vi "gyro -- async pll monitor V1.vi"(11 "pll monitor event pair IN":T6) -> ()   [LabVIEW 2020]
uses:
  lorentzian.ctl
  circle corners.ctl
  show-win- control.ctl
  server talk-to-back pair.ctl
  server talkback message type.ctl
  server talkto message type.ctl
  interpolation state - real.ctl
  pll internal user event action.ctl
  launch items list.ctl
  que event bag action.ctl
  agregator -- action.ctl
  interpolation state - complex.ctl
  publisher action.ctl
  cursor action.ctl
  four-corner circle transformation.ctl
  linear interpolation iiii- complex.vi
  replace cursor action stack.vi
  Q -- range multiplier -- real -- V2.vi
  Q - not nan and gtr than zero - Real.vi
  Q - not nan -- real.vi
  Q -- check range -- i -- real.vi
  array - smart min max.vi
  linear interpolation - real.vi
  draw a circle.vi
  draw a complex arrow.vi
  generate linear region.vi
  draw a complex line.vi
panel:
  in  "all 3":T1(tab)
  in  "Reset lore :q":bool
  in  "Tab Control":enum32{"PID", "hist", "params"}(tab)
  out "Plot: complex plane":cluster{dbl[], dbl[]}[](graph)=[{[0.0, 0.0, 0.0, 0.0, 0.0, 0.0, 0.0, 0.0, 0.0, 0.0, 0.0, 0.0, 0.0, 0.0, 0.0, 0.0, 0.0, 0.0, 0.0, 0.0, 0.0, 0.0, 0.0, 0.0, 0.0, 0.0, 0.0, 0.0, 0.0, 0.0, 0.0, 0.0, 0.0, 0.0, 0.0, 0.0, 0.0, 0.0, 0.0, 0.0, 0.0, 0.0, 0.0, 0.0, 0.0, 0.0, 0.0, 0.0, 0.0, 0.0, 0.0, 0.0, 0.0, 0.0, 0.0, 0.0, 0.0, 0.0, 0.0, 0.0, 0.0, 0.0, 0.0, 0.0, 0.0, 0.0, 0.0, 0.0, 0.0, 0.0, 0.0, 0.0, 0.0, 0.0, 0.0, 0.0, 0.0, 0.0, 0.0, 0.0, 0.0, 0.0, 0.0, 0.0, 0.0, 0.0, 0.0, 0.0, 0.0, 0.0, 0.0, 0.0, 0.0, 0.0, 0.0, 0.0, 0.0, 0.0, 0.0, 0.0, 0.0, 0.0, 0.0, 0.0, 0.0, 0.0, 0.0, 0.0, 0.0, 0.0, 0.0, 0.0, 0.0, 0.0, 0.0, 0.0, 0.0, 0.0, 0.0, 0.0, 0.0, 0.0, 0.0, 0.0, 0.0, 0.0, 0.0, 0.0, 0.0, 0.0, 0.0, 0.0, 0.0, 0.0, 0.0, 0.0, 0.0, 0.0, 0.0, 0.0, 0.0, 0.0, 0.0, 0.0, 0.0, 0.0, 0.0, 0.0, 0.0, 0.0], [0.0, 0.0, 0.0, 0.0, 0.0, 0.0, 0.0, 0.0, 0.0, 0.0, 0.0, 0.0, 0.0, 0.0, 0.0, 0.0, 0.0, 0.0, 0.0, 0.0, 0.0, 0.0, 0.0, 0.0, 0.0, 0.0, 0.0, 0.0, 0.0, 0.0, 0.0, 0.0, 0.0, 0.0, 0.0, 0.0, 0.0, 0.0, 0.0, 0.0, 0.0, 0.0, 0.0, 0.0, 0.0, 0.0, 0.0, 0.0, 0.0, 0.0, 0.0, 0.0, 0.0, 0.0, 0.0, 0.0, 0.0, 0.0, 0.0, 0.0, 0.0, 0.0, 0.0, 0.0, 0.0, 0.0, 0.0, 0.0, 0.0, 0.0, 0.0, 0.0, 0.0, 0.0, 0.0, 0.0, 0.0, 0.0, 0.0, 0.0, 0.0, 0.0, 0.0, 0.0, 0.0, 0.0, 0.0, 0.0, 0.0, 0.0, 0.0, 0.0, 0.0, 0.0, 0.0, 0.0, 0.0, 0.0, 0.0, 0.0, 0.0, 0.0, 0.0, 0.0, 0.0, 0.0, 0.0, 0.0, 0.0, 0.0, 0.0, 0.0, 0.0, 0.0, 0.0, 0.0, 0.0, 0.0, 0.0, 0.0, 0.0, 0.0, 0.0, 0.0, 0.0, 0.0, 0.0, 0.0, 0.0, 0.0, 0.0, 0.0, 0.0, 0.0, 0.0, 0.0, 0.0, 0.0, 0.0, 0.0, 0.0, 0.0, 0.0, 0.0, 0.0, 0.0, 0.0, 0.0, 0.0, 0.0]}, {[0.0, 0.0, 0.0, 0.0, 0.0, 0.0, 0.0, 0.0, 0.0, 0.0, 0.0, 0.0, 0.0, 0.0, 0.0, 0.0, 0.0, 0.0, 0.0, 0.0], [0.0, 0.0, 0.0, 0.0, 0.0, 0.0, 0.0, 0.0, 0.0, 0.0, 0.0, 0.0, 0.0, 0.0, 0.0, 0.0, 0.0, 0.0, 0.0, 0.0]}, {[0.0, 0.0, 0.0, 0.0, 0.0, 0.0, 0.0, 0.0, 0.0, 0.0, 0.0, 0.0, 0.0, 0.0, 0.0, 0.0, 0.0, 0.0, 0.0, 0.0], [0.0, 0.0, 0.0, 0.0, 0.0, 0.0, 0.0, 0.0, 0.0, 0.0, 0.0, 0.0, 0.0, 0.0, 0.0, 0.0, 0.0, 0.0, 0.0, 0.0]}, {[0.0, 0.0, 0.0, 0.0, 0.0, 0.0, 0.0, 0.0, 0.0, 0.0, 0.0, 0.0, 0.0, 0.0, 0.0, 0.0, 0.0, 0.0, 0.0, 0.0], [0.0, 0.0, 0.0, 0.0, 0.0, 0.0, 0.0, 0.0, 0.0, 0.0, 0.0, 0.0, 0.0, 0.0, 0.0, 0.0, 0.0, 0.0, 0.0, 0.0]}, {[0.0, 0.0, 0.0, 0.0, 0.0, 0.0, 0.0, 0.0, 0.0, 0.0, 0.0, 0.0, 0.0, 0.0, 0.0, 0.0, 0.0, 0.0, 0.0, 0.0], [0.0, 0.0, 0.0, 0.0, 0.0, 0.0, 0.0, 0.0, 0.0, 0.0, 0.0, 0.0, 0.0, 0.0, 0.0, 0.0, 0.0, 0.0, 0.0, 0.0]}, {[0.0, 0.0, 0.0, 0.0, 0.0, 0.0, 0.0, 0.0, 0.0, 0.0, 0.0, 0.0, 0.0, 0.0, 0.0, 0.0, 0.0, 0.0, 0.0, 0.0], [0.0, 0.0, 0.0, 0.0, 0.0, 0.0, 0.0, 0.0, 0.0, 0.0, 0.0, 0.0, 0.0, 0.0, 0.0, 0.0, 0.0, 0.0, 0.0, 0.0]}, {[0.0, 0.0, 0.0, 0.0, 0.0, 0.0, 0.0, 0.0, 0.0, 0.0, 0.0, 0.0, 0.0, 0.0, 0.0, 0.0, 0.0, 0.0, 0.0, 0.0], [0.0, 0.0, 0.0, 0.0, 0.0, 0.0, 0.0, 0.0, 0.0, 0.0, 0.0, 0.0, 0.0, 0.0, 0.0, 0.0, 0.0, 0.0, 0.0, 0.0]}, {[0.0, 0.0, 0.0, 0.0, 0.0, 0.0, 0.0, 0.0, 0.0, 0.0, 0.0, 0.0, 0.0, 0.0, 0.0, 0.0, 0.0, 0.0, 0.0, 0.0], [0.0, 0.0, 0.0, 0.0, 0.0, 0.0, 0.0, 0.0, 0.0, 0.0, 0.0, 0.0, 0.0, 0.0, 0.0, 0.0, 0.0, 0.0, 0.0, 0.0]}, {[0.0, 0.0, 0.0, 0.0, 0.0, 0.0, 0.0, 0.0, 0.0, 0.0, 0.0, 0.0, 0.0, 0.0, 0.0, 0.0, 0.0, 0.0, 0.0, 0.0], [0.0, 0.0, 0.0, 0.0, 0.0, 0.0, 0.0, 0.0, 0.0, 0.0, 0.0, 0.0, 0.0, 0.0, 0.0, 0.0, 0.0, 0.0, 0.0, 0.0]}, {[0.0, 0.0, 0.0, 0.0, 0.0, 0.0, 0.0, 0.0, 0.0, 0.0, 0.0, 0.0, 0.0, 0.0, 0.0, 0.0, 0.0, 0.0, 0.0, 0.0], [0.0, 0.0, 0.0, 0.0, 0.0, 0.0, 0.0, 0.0, 0.0, 0.0, 0.0, 0.0, 0.0, 0.0, 0.0, 0.0, 0.0, 0.0, 0.0, 0.0]}, {[0.03998951555184836, 0.03997962657760714, 0.0399499770035046, 0.039900618844968684, 0.03983163869298151, 0.03974315756216925, 0.03963533067850146, 0.039508347206971904, 0.03936242991973892, 0.03919783480530734, 0.039014850619437685, 0.038813798378570394, 0.038595030796653974, 0.03835893166636482, 0.0381059151858045, 0.03783642523185548, 0.03755093458147029, 0.03724994408226008, 0.03693398177383773, 0.036603601961456914, 0.036259384243572376, 0.035901932495027246, 0.035531873807651396, 0.03514985739012926, 0.034756553429067236, 0.034352651913258606, 0.03393886142320875, 0.03351590788804418, 0.03308453331198614, 0.032645494472623104, 0.032199561593265716, 0.03174751699171339, 0.03129015370780302, 0.030828274112147683, 0.0303626884985059, 0.02989421366225105, 0.02942367146743474, 0.02895188740495799, 0.028479689144379698, 0.02800790508190295, 0.027537362887086643, 0.02706888805083179, 0.026603302437190005, 0.026141422841534666, 0.0256840595576243, 0.02523201495607197, 0.024786082076714587, 0.024347043237351554, 0.023915668661293514, 0.023492715126128938, 0.023078924636079086, 0.02267502312027045, 0.022281719159208423, 0.021899702741686292, 0.021529644054310442, 0.021172192305765312, 0.02082797458788077, 0.020497594775499964, 0.020181632467077607, 0.0198806419678674, 0.019595151317482205, 0.019325661363533187, 0.01907264488297286, 0.01883654575268371, 0.01861777817076729, 0.018416725929900006, 0.018233741744030342, 0.018069146629598767, 0.017923229342365784, 0.017796245870836228, 0.017688418987168435, 0.017599937856356183, 0.017530957704369, 0.017481599545833094, 0.017451949971730545, 0.017442060997489323, 0.017451949971730545, 0.01748159954583309, 0.017530957704369, 0.01759993785635618, 0.017688418987168435, 0.017796245870836225, 0.01792322934236578, 0.018069146629598763, 0.018233741744030342, 0.0184167259299, 0.01861777817076729, 0.01883654575268371, 0.019072644882972854, 0.01932566136353318, 0.019595151317482202, 0.019880641967867395, 0.020181632467077604, 0.020497594775499957, 0.020827974587880767, 0.02117219230576531, 0.02152964405431043, 0.021899702741686285, 0.02228171915920842, 0.022675023120270445, 0.02307892463607908, 0.02349271512612893, 0.023915668661293507, 0.024347043237351547, 0.02478608207671458, 0.025232014956071965, 0.025684059557624296, 0.026141422841534655, 0.02660330243718999, 0.02706888805083178, 0.027537362887086633, 0.02800790508190294, 0.028479689144379688, 0.028951887404957983, 0.02942367146743473, 0.029894213662251038, 0.03036268849850589, 0.03082827411214768, 0.03129015370780302, 0.03174751699171338, 0.032199561593265716, 0.03264549447262309, 0.033084533311986124, 0.033515907888044164, 0.03393886142320874, 0.03435265191325859, 0.03475655342906723, 0.035149857390129255, 0.03553187380765139, 0.03590193249502724, 0.03625938424357237, 0.036603601961456914, 0.03693398177383772, 0.037249944082260074, 0.03755093458147028, 0.03783642523185548, 0.038105915185804494, 0.03835893166636482, 0.03859503079665397, 0.038813798378570394, 0.03901485061943768, 0.039197834805307336, 0.039362429919738914, 0.0395083472069719, 0.03963533067850146, 0.03974315756216925, 0.0398316386929815, 0.039900618844968684, 0.03994997700350459, 0.03997962657760714], [0.0009917204990441924, 0.0014638151987407945, 0.001935081683915272, 0.002404693193015201, 0.002871825867878557, 0.003335660199060881, 0.003795382463533313, 0.004250186152229294, 0.0046992733849355196, 0.005141856310044955, 0.005577158486716272, 0.006004416247014914, 0.006422880035646153, 0.006831815724929783, 0.007230505902709515, 0.007618251130937694, 0.007994371172727291, 0.00835820618571856, 0.008709117879666748, 0.009046490636220072, 0.009369732588923506, 0.009678276661553653, 0.009971581562963142, 0.010249132736689223, 0.010510443263660659, 0.010755054716419228, 0.01098253796335726, 0.011192493921560302, 0.011384554256934151, 0.01155838203038802, 0.011713672288940196, 0.011850152600709193, 0.011967583532851852, 0.01206575907160989, 0.012144506983728055, 0.012203689118609773, 0.012243201650680236, 0.012262975261531743, 0.012262975261531743, 0.012243201650680236, 0.012203689118609773, 0.012144506983728057, 0.01206575907160989, 0.011967583532851852, 0.011850152600709195, 0.011713672288940196, 0.011558382030388021, 0.011384554256934153, 0.011192493921560305, 0.010982537963357263, 0.01075505471641923, 0.01051044326366066, 0.010249132736689225, 0.009971581562963143, 0.009678276661553659, 0.00936973258892351, 0.009046490636220076, 0.008709117879666751, 0.008358206185718564, 0.007994371172727293, 0.007618251130937694, 0.00723050590270952, 0.006831815724929786, 0.006422880035646157, 0.0060044162470149175, 0.005577158486716275, 0.005141856310044959, 0.004699273384935521, 0.0042501861522293, 0.0037953824635333184, 0.0033356601990608852, 0.0028718258678785613, 0.0024046931930152044, 0.0019350816839152748, 0.0014638151987407966, 0.0009917204990441987, 0.0005196257993475959, 4.835931417311785e-05, -0.0004212521949268119, -0.0008883848697901688, -0.001352219200972493, -0.0018119414654449257, -0.002266745154140903, -0.0027158323868471295, -0.0031584153119565664, -0.003593717488627883, -0.004020975248926525, -0.004439439037557766, -0.004848374726841395, -0.005247064904621124, -0.005634810132849303, -0.006010930174638902, -0.006374765187630173, -0.0067256768815783605, -0.007063049638131685, -0.007386291590835118, -0.007694835663465264, -0.007988140564874752, -0.008265691738600834, -0.00852700226557227, -0.00877161371833084, -0.008999096965268873, -0.009209052923471916, -0.009401113258845765, -0.009574941032299633, -0.009730231290851809, -0.009866711602620808, -0.009984142534763464, -0.010082318073521503, -0.01016106598563967, -0.010220248120521387, -0.01025976065259185, -0.010279534263443357, -0.010279534263443357, -0.010259760652591852, -0.01022024812052139, -0.010161065985639671, -0.010082318073521505, -0.009984142534763468, -0.00986671160262081, -0.00973023129085181, -0.009574941032299639, -0.00940111325884577, -0.009209052923471921, -0.00899909696526888, -0.008771613718330847, -0.008527002265572278, -0.008265691738600842, -0.007988140564874761, -0.007694835663465273, -0.007386291590835125, -0.007063049638131692, -0.0067256768815783675, -0.00637476518763018, -0.00601093017463891, -0.00563481013284931, -0.005247064904621139, -0.004848374726841407, -0.004439439037557778, -0.004020975248926537, -0.003593717488627896, -0.0031584153119565794, -0.0027158323868471425, -0.0022667451541409167, -0.0018119414654449348, -0.001352219200972502, -0.0008883848697901777, -0.000421252194926821, 4.835931417310874e-05, 0.0005196257993475868]}, {[0.018500144394306906, 0.019575475329081847, 0.020650806263856788, 0.02172613719863173, 0.02280146813340667, 0.02387679906818161, 0.02495213000295655, 0.026027460937731492, 0.027102791872506433, 0.028178122807281374, 0.029253453742056314, 0.030328784676831255, 0.03140411561160619, 0.03247944654638114, 0.03355477748115608, 0.03463010841593102, 0.035705439350705956, 0.0367807702854809, 0.037856101220255844, 0.03893143215503078], [-0.0037766698823995634, -0.003274734052773905, -0.0027727982231482463, -0.002270862393522588, -0.0017689265638969297, -0.001266990734271271, -0.0007650549046456126, -0.00026311907501995425, 0.00023881675460570408, 0.0007407525842313633, 0.0012426884138570216, 0.0017446242434826808, 0.0022465600731083383, 0.0027484959027339975, 0.003250431732359655, 0.003752367561985314, 0.004254303391610972, 0.004756239221236632, 0.00525817505086229, 0.005760110880487949]}, {[0.03893143215503078, 0.03887322269693558, 0.03881501323884037, 0.03875680378074517, 0.038698594322649965, 0.03864038486455476, 0.03858217540645956, 0.03852396594836435, 0.03846575649026915, 0.038407547032173944, 0.03834933757407875, 0.03829112811598354, 0.03823291865788834, 0.038174709199793135, 0.03811649974169793, 0.038058290283602726, 0.03800008082550752, 0.03794187136741232, 0.037883661909317114, 0.03782545245122191], [0.005760110880487949, 0.0057486065561215376, 0.005737102231755127, 0.005725597907388716, 0.005714093583022305, 0.0057025892586558945, 0.005691084934289483, 0.005679580609923073, 0.005668076285556662, 0.005656571961190251, 0.00564506763682384, 0.005633563312457429, 0.005622058988091018, 0.005610554663724608, 0.0055990503393581964, 0.005587546014991786, 0.005576041690625375, 0.005564537366258964, 0.005553033041892553, 0.005541528717526142]}, {[0.03893143215503078, 0.038885231477990216, 0.03883903080094966, 0.03879283012390909, 0.038746629446868526, 0.03870042876982797, 0.0386542280927874, 0.038608027415746836, 0.03856182673870628, 0.03851562606166571, 0.038469425384625146, 0.03842322470758458, 0.03837702403054402, 0.038330823353503456, 0.03828462267646289, 0.03823842199942233, 0.038192221322381766, 0.0381460206453412, 0.03809981996830064, 0.038053619291260075], [0.005760110880487949, 0.005722879335638743, 0.005685647790789537, 0.005648416245940331, 0.005611184701091125, 0.00557395315624192, 0.005536721611392714, 0.005499490066543508, 0.0054622585216943026, 0.0054250269768450965, 0.00538779543199589, 0.005350563887146684, 0.005313332342297479, 0.005276100797448273, 0.005238869252599067, 0.005201637707749862, 0.0051644061629006555, 0.005127174618051449, 0.005089943073202244, 0.005052711528353038]}, {[0.023947397893225086, 0.024449333722850745, 0.024951269552476403, 0.02545320538210206, 0.02595514121172772, 0.026457077041353378, 0.026959012870979036, 0.027460948700604695, 0.027962884530230353, 0.028464820359856015, 0.02896675618948167, 0.02946869201910733, 0.029970627848732986, 0.030472563678358648, 0.030974499507984303, 0.031476435337609965, 0.03197837116723562, 0.03248030699686128, 0.03298224282648694, 0.0334841786561126], [0.01120736437940613, 0.01013203344463119, 0.009056702509856249, 0.007981371575081308, 0.006906040640306367, 0.005830709705531427, 0.004755378770756486, 0.003680047835981545, 0.002604716901206604, 0.0015293859664316633, 0.00045405503165672247, -0.0006212759031182184, -0.0016966068378931592, -0.0027719377726681, -0.003847268707443041, -0.004922599642217982, -0.0059979305769929225, -0.007073261511767863, -0.008148592446542804, -0.009223923381317745]}, {[0.0334841786561126, 0.03347267433174619, 0.033461170007379776, 0.033449665683013365, 0.03343816135864695, 0.03342665703428054, 0.03341515270991413, 0.03340364838554772, 0.03339214406118131, 0.0333806397368149, 0.03336913541244849, 0.03335763108808208, 0.03334612676371567, 0.03333462243934926, 0.03332311811498285, 0.03331161379061644, 0.033300109466250026, 0.033288605141883615, 0.033277100817517204, 0.03326559649315079], [-0.009223923381317745, -0.00916571392322254, -0.009107504465127338, -0.009049295007032134, -0.00899108554893693, -0.008932876090841728, -0.008874666632746523, -0.00881645717465132, -0.008758247716556117, -0.008700038258460913, -0.008641828800365708, -0.008583619342270504, -0.008525409884175302, -0.008467200426080098, -0.008408990967984893, -0.008350781509889691, -0.008292572051794487, -0.008234362593699283, -0.00817615313560408, -0.008117943677508876]}, {[0.0334841786561126, 0.03344694711126339, 0.033409715566414186, 0.03337248402156498, 0.033335252476715774, 0.03329802093186657, 0.03326078938701736, 0.033223557842168155, 0.03318632629731895, 0.03314909475246974, 0.033111863207620544, 0.03307463166277134, 0.03303740011792213, 0.033000168573072926, 0.03296293702822372, 0.032925705483374514, 0.03288847393852531, 0.0328512423936761, 0.032814010848826895, 0.03277677930397769], [-0.009223923381317745, -0.009177722704277181, -0.009131522027236619, -0.009085321350196055, -0.00903912067315549, -0.008992919996114929, -0.008946719319074365, -0.0089005186420338, -0.008854317964993239, -0.008808117287952675, -0.00876191661091211, -0.008715715933871547, -0.008669515256830984, -0.00862331457979042, -0.008577113902749857, -0.008530913225709294, -0.00848471254866873, -0.008438511871628166, -0.008392311194587604, -0.00834611051754704]}, {[0.02803692515719442, 0.027033053497943105, 0.026029181838691788, 0.02502531017944047, 0.024021438520189155, 0.023017566860937838, 0.02201369520168652, 0.021009823542435205, 0.020005951883183888, 0.019002080223932568, 0.01799820856468125, 0.01699433690542993, 0.015990465246178618, 0.0149865935869273, 0.013982721927675985, 0.012978850268424666, 0.011974978609173351, 0.010971106949922031, 0.009967235290670715, 0.008963363631419398], [-0.02420795764312344, -0.022057295773573557, -0.019906633904023675, -0.017755972034473794, -0.015605310164923912, -0.01345464829537403, -0.011303986425824149, -0.009153324556274267, -0.0070026626867243855, -0.004852000817174504, -0.002701338947624622, -0.0005506770780747405, 0.0015999847914751411, 0.0037506466610250228, 0.005901308530574904, 0.008051970400124786, 0.010202632269674668, 0.01235329413922455, 0.014503956008774431, 0.016654617878324313]}, {[0.008963363631419396, 0.008986372280152219, 0.00900938092888504, 0.009032389577617862, 0.009055398226350684, 0.009078406875083505, 0.009101415523816327, 0.009124424172549148, 0.00914743282128197, 0.009170441470014792, 0.009193450118747613, 0.009216458767480435, 0.009239467416213258, 0.009262476064946078, 0.0092854847136789, 0.009308493362411721, 0.009331502011144544, 0.009354510659877366, 0.009377519308610187, 0.00940052795734301], [0.016654617878324313, 0.016538198962133904, 0.0164217800459435, 0.01630536112975309, 0.016188942213562683, 0.016072523297372274, 0.01595610438118187, 0.01583968546499146, 0.015723266548801053, 0.015606847632610646, 0.01549042871642024, 0.015374009800229831, 0.015257590884039425, 0.015141171967849018, 0.01502475305165861, 0.014908334135468203, 0.014791915219277795, 0.014675496303087388, 0.01455907738689698, 0.014442658470706573]}, {[0.008963363631419396, 0.009037826721117808, 0.009112289810816219, 0.009186752900514631, 0.009261215990213043, 0.009335679079911454, 0.009410142169609866, 0.009484605259308276, 0.009559068349006689, 0.0096335314387051, 0.009707994528403511, 0.009782457618101923, 0.009856920707800336, 0.009931383797498746, 0.010005846887197158, 0.01008030997689557, 0.010154773066593981, 0.010229236156292393, 0.010303699245990804, 0.010378162335689216], [0.016654617878324313, 0.016562216524243185, 0.01646981517016206, 0.016377413816080932, 0.016285012461999804, 0.01619261110791868, 0.016100209753837552, 0.016007808399756424, 0.0159154070456753, 0.015823005691594172, 0.015730604337513044, 0.015638202983431916, 0.015545801629350792, 0.015453400275269664, 0.015360998921188538, 0.015268597567107411, 0.015176196213026284, 0.015083794858945157, 0.01499139350486403, 0.014898992150782903]}]
  out "Plot: complex- hist":cluster{dbl[], dbl[]}[](graph)=[{[-9.526305317469014e-05, -9.526305317469014e-05, -9.526305317469014e-05, -9.526305317469014e-05, -9.526305317469014e-05, -9.526305317469014e-05, -9.526305317469014e-05, -9.526305317469014e-05, -9.526305317469014e-05, -9.526305317469014e-05, -9.526305317469014e-05, -9.526305317469014e-05, -9.496573362823372e-05, -9.462272279446522e-05, -9.456910422622903e-05, -9.455599564968666e-05, -9.455599564968666e-05, -9.455599564968666e-05, -9.455599564968666e-05, -9.455599564968666e-05, -9.455599564968666e-05, -9.530610879315279e-05, -9.530610879315279e-05, -9.634850628222362e-05, -9.634850628222362e-05, -9.634850628222362e-05, -9.634850628222362e-05, -9.634850628222362e-05, -9.634850628222362e-05, -9.634850628222362e-05, -0.00010067313796781224, -0.00010168181201432396, -0.00010343088718200523, -0.00010398871218266516, -0.00010398871218266516, -0.00010398871218266516, -0.00010398871218266516, -0.00010398871218266516, -0.00010398871218266516, -0.00010398871218266516, -0.00010398871218266516, -0.00010398871218266516, -0.00011483545491618031, -0.00011483545491618031, -0.00011483545491618031, -0.00011483545491618031, -0.00011483545491618031, -0.00011483545491618031, -0.00011483545491618031, -0.00011483545491618031], [7.970920146417072e-05, 7.970920146417072e-05, 7.970920146417072e-05, 7.970920146417072e-05, 7.970920146417072e-05, 7.970920146417072e-05, 7.970920146417072e-05, 7.970920146417072e-05, 7.970920146417072e-05, 7.970920146417072e-05, 7.970920146417072e-05, 7.970920146417072e-05, 7.992857617299889e-05, 8.004706678063113e-05, 8.0440222108718e-05, 8.032807976592085e-05, 8.032807976592085e-05, 8.032807976592085e-05, 8.032807976592085e-05, 8.032807976592085e-05, 8.032807976592085e-05, 8.12855651877623e-05, 8.12855651877623e-05, 8.097547218826884e-05, 8.097547218826884e-05, 8.097547218826884e-05, 8.097547218826884e-05, 8.097547218826884e-05, 8.097547218826884e-05, 8.097547218826884e-05, 8.470777605978184e-05, 8.527717057334149e-05, 8.650804581518505e-05, 8.815252786351578e-05, 8.815252786351578e-05, 8.815252786351578e-05, 8.815252786351578e-05, 8.815252786351578e-05, 8.815252786351578e-05, 8.815252786351578e-05, 8.815252786351578e-05, 8.815252786351578e-05, 9.872168338494033e-05, 9.872168338494033e-05, 9.872168338494033e-05, 9.872168338494033e-05, 9.872168338494033e-05, 9.872168338494033e-05, 9.872168338494033e-05, 9.872168338494033e-05]}, {[3.818876044553316e-06, 3.7612071619776832e-06, 3.588301685066841e-06, 3.300462948780953e-06, 2.8981959200717497e-06, 2.3822063119988216e-06, 1.7533993456691853e-06, 1.0128781621718285e-06, 1.6194188729338013e-07, -7.979166475899173e-07, -1.8650135244457675e-06, -3.037476692750206e-06, -4.313249253700366e-06, -5.690093068713917e-06, -7.1655926858846405e-06, -8.737159577505894e-06, -1.0402036681227744e-05, -1.2157303236881222e-05, -1.3999879910484142e-05, -1.592653419643923e-05, -1.79338860884474e-05, -2.001841400918731e-05, -2.2176460988358644e-05, -2.440424107825063e-05, -2.6697845995580853e-05, -2.9053251977952116e-05, -3.146632684289902e-05, -3.3932837237140076e-05, -3.6448456063317944e-05, -3.900877007119849e-05, -4.1609287600011325e-05, -4.4245446458349125e-05, -4.691262192780158e-05, -4.9606134876282945e-05, -5.232125996681972e-05, -5.505323394739742e-05, -5.779726400732312e-05, -6.054853618544401e-05, -6.330222381547109e-05, -6.605349599359198e-05, -6.879752605351768e-05, -7.152950003409537e-05, -7.424462512463216e-05, -7.693813807311352e-05, -7.960531354256597e-05, -8.224147240090377e-05, -8.484198992971662e-05, -8.740230393759715e-05, -8.991792276377502e-05, -9.238443315801609e-05, -9.479750802296298e-05, -9.715291400533426e-05, -9.944651892266448e-05, -0.00010167429901255647, -0.00010383234599172779, -0.00010591687391246771, -0.00010792422580447587, -0.00010985088009043097, -0.00011169345676403388, -0.00011344872331968736, -0.00011511360042340923, -0.00011668516731503045, -0.00011816066693220119, -0.00011953751074721475, -0.0001208132833081649, -0.00012198574647646935, -0.0001230528433533252, -0.0001240127018882085, -0.00012486363816308695, -0.0001256041593465843, -0.00012623296631291396, -0.00012674895592098688, -0.00012715122294969607, -0.00012743906168598198, -0.00012761196716289282, -0.00012766963604546842, -0.00012761196716289282, -0.00012743906168598198, -0.00012715122294969607, -0.00012674895592098688, -0.00012623296631291396, -0.00012560415934658432, -0.00012486363816308695, -0.00012401270188820853, -0.00012305284335332523, -0.00012198574647646936, -0.00012081328330816493, -0.00011953751074721476, -0.00011816066693220122, -0.00011668516731503051, -0.00011511360042340925, -0.00011344872331968739, -0.0001116934567640339, -0.000109850880090431, -0.00010792422580447591, -0.00010591687391246773, -0.00010383234599172784, -0.0001016742990125565, -9.944651892266452e-05, -9.715291400533429e-05, -9.479750802296303e-05, -9.238443315801612e-05, -8.991792276377506e-05, -8.740230393759719e-05, -8.484198992971665e-05, -8.22414724009038e-05, -7.9605313542566e-05, -7.69381380731136e-05, -7.424462512463222e-05, -7.152950003409544e-05, -6.879752605351773e-05, -6.605349599359204e-05, -6.330222381547115e-05, -6.054853618544405e-05, -5.779726400732316e-05, -5.505323394739747e-05, -5.232125996681976e-05, -4.960613487628297e-05, -4.691262192780161e-05, -4.424544645834915e-05, -4.160928760001134e-05, -3.900877007119856e-05, -3.644845606331801e-05, -3.393283723714014e-05, -3.146632684289907e-05, -2.905325197795217e-05, -2.66978459955809e-05, -2.4404241078250677e-05, -2.2176460988358678e-05, -2.0018414009187342e-05, -1.7933886088447427e-05, -1.5926534196439257e-05, -1.3999879910484162e-05, -1.2157303236881242e-05, -1.0402036681227757e-05, -8.7371595775059e-06, -7.165592685884681e-06, -5.690093068713951e-06, -4.3132492537004e-06, -3.037476692750233e-06, -1.8650135244457946e-06, -7.979166475899309e-07, 1.6194188729336657e-07, 1.012878162171815e-06, 1.7533993456691853e-06, 2.3822063119988216e-06, 2.8981959200717497e-06, 3.300462948780953e-06, 3.588301685066841e-06, 3.7612071619776832e-06], [0.00013328633245229232, 0.00013603941615311703, 0.0001387876700096264, 0.0001415262726506931, 0.00014425041963670132, 0.00014695533188816622, 0.0001496362640698634, 0.00015228851291575925, 0.00015490742548013788, 0.00015748840730044888, 0.00016002693045755594, 0.0001625185415192455, 0.0001649588693530602, 0.00016734363279475065, 0.00016966864815889197, 0.00017192983657849, 0.00017412323116069973, 0.00017624498394610346, 0.00017829137265933922, 0.00018025880723923637, 0.00018214383613700304, 0.00018394315237141542, 0.0001856535993303866, 0.00018727217630873675, 0.00018879604377244967, 0.0001902225283401804, 0.0001915491274732744, 0.0001927735138660708, 0.00019389353952878736, 0.00019490723955582442, 0.00019581283557287696, 0.00019660873885680747, 0.00019729355312280615, 0.00019786607697394902, 0.00019832530600885628, 0.0001986704345837536, 0.00019890085722584514, 0.00019901616969551854, 0.00019901616969551854, 0.00019890085722584514, 0.0001986704345837536, 0.00019832530600885628, 0.00019786607697394902, 0.00019729355312280615, 0.00019660873885680747, 0.00019581283557287696, 0.00019490723955582442, 0.0001938935395287874, 0.00019277351386607082, 0.0001915491274732744, 0.0001902225283401804, 0.00018879604377244967, 0.00018727217630873675, 0.00018565359933038662, 0.00018394315237141545, 0.00018214383613700307, 0.00018025880723923637, 0.00017829137265933922, 0.00017624498394610348, 0.00017412323116069973, 0.00017192983657849, 0.000169668648158892, 0.00016734363279475065, 0.00016495886935306023, 0.00016251854151924552, 0.00016002693045755596, 0.0001574884073004489, 0.00015490742548013788, 0.00015228851291575928, 0.00014963626406986344, 0.00014695533188816625, 0.00014425041963670135, 0.00014152627265069312, 0.0001387876700096264, 0.00013603941615311706, 0.00013328633245229235, 0.00013053324875146764, 0.0001277849948949583, 0.00012504639225389158, 0.00012232224526788335, 0.00011961733301641843, 0.00011693640083472126, 0.00011428415198882542, 0.0001116652394244468, 0.00010908425760413579, 0.00010654573444702874, 0.00010405412338533918, 0.00010161379555152444, 9.922903210983402e-05, 9.69040167456927e-05, 9.464282832609468e-05, 9.244943374388495e-05, 9.032768095848119e-05, 8.828129224524545e-05, 8.631385766534829e-05, 8.44288287675816e-05, 8.262951253316924e-05, 8.091906557419806e-05, 7.930048859584792e-05, 7.777662113213499e-05, 7.635013656440427e-05, 7.502353743131027e-05, 7.379915103851385e-05, 7.267912537579728e-05, 7.166542534876021e-05, 7.07598293317077e-05, 6.996392604777719e-05, 6.927911178177851e-05, 6.870658793063563e-05, 6.824735889572837e-05, 6.790223032083105e-05, 6.76718076787395e-05, 6.755649520906611e-05, 6.755649520906611e-05, 6.76718076787395e-05, 6.790223032083104e-05, 6.824735889572836e-05, 6.870658793063562e-05, 6.92791117817785e-05, 6.996392604777719e-05, 7.075982933170768e-05, 7.166542534876019e-05, 7.267912537579724e-05, 7.379915103851382e-05, 7.502353743131023e-05, 7.635013656440423e-05, 7.777662113213495e-05, 7.930048859584787e-05, 8.091906557419801e-05, 8.262951253316918e-05, 8.442882876758158e-05, 8.631385766534825e-05, 8.828129224524542e-05, 9.032768095848116e-05, 9.244943374388492e-05, 9.464282832609465e-05, 9.690401674569261e-05, 9.922903210983394e-05, 0.00010161379555152437, 0.00010405412338533911, 0.00010654573444702866, 0.00010908425760413571, 0.00011166523942444672, 0.00011428415198882535, 0.0001169364008347212, 0.00011961733301641839, 0.0001223222452678833, 0.00012504639225389153, 0.00012778499489495826, 0.0001305332487514676]}, {[3.628480178228017e-06, -3.271926156370463e-06, -1.0172332490968943e-05, -1.7072738825567422e-05, -2.3973145160165903e-05, -3.087355149476438e-05, -3.777395782936286e-05, -4.467436416396134e-05, -5.157477049855982e-05, -5.8475176833158303e-05, -6.537558316775678e-05, -7.227598950235527e-05, -7.917639583695374e-05, -8.607680217155223e-05, -9.29772085061507e-05, -9.987761484074919e-05, -0.00010677802117534766, -0.00011367842750994615, -0.00012057883384454462, -0.00012747924017914312], [0.00013828619430891303, 0.0001377598930608477, 0.00013723359181278235, 0.00013670729056471703, 0.00013618098931665167, 0.00013565468806858635, 0.000135128386820521, 0.00013460208557245567, 0.00013407578432439034, 0.00013354948307632499, 0.00013302318182825966, 0.0001324968805801943, 0.00013197057933212898, 0.00013144427808406365, 0.0001309179768359983, 0.00013039167558793297, 0.00012986537433986762, 0.0001293390730918023, 0.00012881277184373694, 0.00012828647059567161]}, {[-0.00012747924017914312, -0.0001271379440244435, -0.00012679664786974387, -0.00012645535171504425, -0.00012611405556034463, -0.00012577275940564502, -0.00012543146325094537, -0.00012509016709624576, -0.00012474887094154614, -0.00012440757478684653, -0.00012406627863214688, -0.00012372498247744727, -0.00012338368632274765, -0.00012304239016804804, -0.0001227010940133484, -0.00012235979785864878, -0.00012201850170394916, -0.00012167720554924953, -0.00012133590939454991, -0.00012099461323985029], [0.00012828647059567161, 0.00012822947554103566, 0.0001281724804863997, 0.00012811548543176373, 0.00012805849037712778, 0.00012800149532249183, 0.00012794450026785587, 0.00012788750521321992, 0.00012783051015858394, 0.000127773515103948, 0.00012771652004931204, 0.0001276595249946761, 0.0001276025299400401, 0.00012754553488540416, 0.0001274885398307682, 0.00012743154477613225, 0.0001273745497214963, 0.00012731755466686032, 0.00012726055961222437, 0.00012720356455758842]}, {[-0.00012747924017914312, -0.00012715053574649993, -0.0001268218313138567, -0.0001264931268812135, -0.00012616442244857027, -0.00012583571801592707, -0.00012550701358328385, -0.00012517830915064065, -0.00012484960471799742, -0.00012452090028535422, -0.00012419219585271102, -0.0001238634914200678, -0.0001235347869874246, -0.00012320608255478137, -0.00012287737812213817, -0.00012254867368949494, -0.00012221996925685174, -0.00012189126482420853, -0.00012156256039156532, -0.0001212338559589221], [0.00012828647059567161, 0.00012839456729972132, 0.00012850266400377103, 0.0001286107607078207, 0.00012871885741187042, 0.00012882695411592013, 0.00012893505081996984, 0.00012904314752401955, 0.00012915124422806923, 0.00012925934093211894, 0.00012936743763616865, 0.00012947553434021836, 0.00012958363104426804, 0.00012969172774831775, 0.00012979982445236746, 0.00012990792115641716, 0.00013001601786046687, 0.00013012411456451655, 0.00013023221126856626, 0.00013034030797261597]}, {[-6.692524185707827e-05, -6.639894060901293e-05, -6.587263936094759e-05, -6.534633811288225e-05, -6.482003686481692e-05, -6.429373561675158e-05, -6.376743436868624e-05, -6.32411331206209e-05, -6.271483187255556e-05, -6.218853062449022e-05, -6.16622293764249e-05, -6.113592812835956e-05, -6.060962688029422e-05, -6.008332563222888e-05, -5.955702438416354e-05, -5.9030723136098205e-05, -5.8504421888032865e-05, -5.7978120639967525e-05, -5.745181939190219e-05, -5.692551814383685e-05], [0.0001988401926309779, 0.0001919397862963794, 0.00018503937996178094, 0.00017813897362718245, 0.00017123856729258396, 0.00016433816095798548, 0.00015743775462338702, 0.00015053734828878853, 0.00014363694195419004, 0.00013673653561959158, 0.0001298361292849931, 0.0001229357229503946, 0.00011603531661579613, 0.00010913491028119764, 0.00010223450394659917, 9.533409761200068e-05, 8.843369127740221e-05, 8.153328494280372e-05, 7.463287860820525e-05, 6.773247227360676e-05]}, {[-5.692551814383685e-05, -5.686852308920089e-05, -5.681152803456494e-05, -5.675453297992898e-05, -5.669753792529302e-05, -5.6640542870657065e-05, -5.658354781602111e-05, -5.6526552761385154e-05, -5.6469557706749195e-05, -5.6412562652113236e-05, -5.6355567597477284e-05, -5.6298572542841325e-05, -5.6241577488205367e-05, -5.618458243356941e-05, -5.6127587378933456e-05, -5.60705923242975e-05, -5.601359726966154e-05, -5.595660221502558e-05, -5.589960716038963e-05, -5.584261210575367e-05], [6.773247227360675e-05, 6.807376842830637e-05, 6.841506458300599e-05, 6.875636073770562e-05, 6.909765689240524e-05, 6.943895304710487e-05, 6.978024920180448e-05, 7.012154535650411e-05, 7.046284151120373e-05, 7.080413766590336e-05, 7.114543382060297e-05, 7.14867299753026e-05, 7.182802613000222e-05, 7.216932228470185e-05, 7.251061843940146e-05, 7.28519145941011e-05, 7.319321074880071e-05, 7.353450690350034e-05, 7.387580305819996e-05, 7.421709921289959e-05]}, {[-5.692551814383685e-05, -5.7033614847886554e-05, -5.7141711551936256e-05, -5.724980825598596e-05, -5.7357904960035666e-05, -5.746600166408537e-05, -5.757409836813507e-05, -5.768219507218477e-05, -5.7790291776234474e-05, -5.7898388480284176e-05, -5.8006485184333885e-05, -5.811458188838359e-05, -5.822267859243329e-05, -5.833077529648299e-05, -5.843887200053269e-05, -5.8546968704582395e-05, -5.86550654086321e-05, -5.8763162112681805e-05, -5.887125881673151e-05, -5.897935552078121e-05], [6.773247227360675e-05, 6.806117670624996e-05, 6.838988113889317e-05, 6.871858557153638e-05, 6.90472900041796e-05, 6.93759944368228e-05, 6.970469886946601e-05, 7.003340330210922e-05, 7.036210773475244e-05, 7.069081216739565e-05, 7.101951660003886e-05, 7.134822103268207e-05, 7.167692546532529e-05, 7.20056298979685e-05, 7.233433433061171e-05, 7.266303876325491e-05, 7.299174319589813e-05, 7.332044762854134e-05, 7.364915206118455e-05, 7.397785649382777e-05]}, {[-6.3712435350134095e-06, -5.318641038882734e-06, -4.266038542752058e-06, -3.213436046621383e-06, -2.160833550490707e-06, -1.1082310543600322e-06, -5.56285582293566e-08, 9.96973937901319e-07, 2.0495764340319955e-06, 3.1021789301626703e-06, 4.154781426293345e-06, 5.2073839224240215e-06, 6.259986418554696e-06, 7.312588914685373e-06, 8.365191410816048e-06, 9.417793906946724e-06, 1.04703964030774e-05, 1.1522998899208077e-05, 1.257560139533875e-05, 1.3628203891469427e-05], [0.00026939391466628416, 0.0002555931019970872, 0.00024179228932789024, 0.0002279914766586933, 0.00021419066398949631, 0.00020038985132029937, 0.00018658903865110242, 0.00017278822598190544, 0.00015898741331270847, 0.00014518660064351152, 0.00013138578797431457, 0.0001175849753051176, 0.00010378416263592065, 8.998334996672367e-05, 7.618253729752673e-05, 6.238172462832975e-05, 4.85809119591328e-05, 3.478009928993583e-05, 2.097928662073888e-05, 7.178473951541904e-06]}, {[1.3628203891469427e-05, 1.374219400074134e-05, 1.3856184110013255e-05, 1.397017421928517e-05, 1.4084164328557083e-05, 1.4198154437828998e-05, 1.4312144547100912e-05, 1.4426134656372826e-05, 1.454012476564474e-05, 1.4654114874916653e-05, 1.4768104984188567e-05, 1.4882095093460481e-05, 1.4996085202732395e-05, 1.511007531200431e-05, 1.5224065421276224e-05, 1.5338055530548138e-05, 1.5452045639820052e-05, 1.5566035749091966e-05, 1.568002585836388e-05, 1.5794015967635795e-05], [7.178473951541904e-06, 7.861066260941151e-06, 8.543658570340397e-06, 9.226250879739644e-06, 9.90884318913889e-06, 1.0591435498538137e-05, 1.1274027807937384e-05, 1.195662011733663e-05, 1.2639212426735877e-05, 1.3321804736135124e-05, 1.400439704553437e-05, 1.4686989354933617e-05, 1.5369581664332864e-05, 1.605217397373211e-05, 1.6734766283131355e-05, 1.7417358592530604e-05, 1.809995090192985e-05, 1.87825432113291e-05, 1.9465135520728344e-05, 2.014772783012759e-05]}, {[1.3628203891469427e-05, 1.3412010483370021e-05, 1.3195817075270614e-05, 1.2979623667171208e-05, 1.2763430259071802e-05, 1.2547236850972395e-05, 1.233104344287299e-05, 1.2114850034773584e-05, 1.1898656626674176e-05, 1.1682463218574771e-05, 1.1466269810475365e-05, 1.1250076402375958e-05, 1.1033882994276552e-05, 1.0817689586177147e-05, 1.0601496178077741e-05, 1.0385302769978334e-05, 1.0169109361878928e-05, 9.95291595377952e-06, 9.736722545680117e-06, 9.52052913758071e-06], [7.178473951541904e-06, 7.835882816828328e-06, 8.49329168211475e-06, 9.150700547401175e-06, 9.8081094126876e-06, 1.0465518277974024e-05, 1.1122927143260446e-05, 1.178033600854687e-05, 1.2437744873833295e-05, 1.3095153739119718e-05, 1.3752562604406142e-05, 1.4409971469692566e-05, 1.506738033497899e-05, 1.5724789200265415e-05, 1.6382198065551837e-05, 1.703960693083826e-05, 1.7697015796124686e-05, 1.8354424661411112e-05, 1.901183352669753e-05, 1.9669242391983957e-05]}]
  in  "hist dt (sec)":dbl=0.1 format="%#_10f"
  in  "plot hist time (sec)":dbl=0.5 format="%#_10f"
  out "fast G (Hz)":dbl=0.9683990629933289 format="%#.4f"
  in  "Reset freq :r":bool
  in  "lorentzian":T2 {"z∞ (V)" format="%#_4p"; "Q" format="%#_4p"; "φ (rad)" format="%#_3p"; "Γ (Hz)" format="%#_5p"; "ω (Hz)" format="%#_9p"; "A (VHz)" format="%#_3p"}
  in  "Toggle PLL :@":bool
  out "fast f (Hz)":dbl=6.9475337429379e-310 format="%#.11f"
  in  "PLL is ON":bool
  in  "publish dt (sec)":dbl=0.05 format="%#_10f"
  in  "lorentzian -- basic":T2={"A (VHz)"=1.0, "ω (Hz)"=1000.0, "Γ (Hz)"=3.0, "φ (rad)"=0.0, "Q"=333.0, "Norm  Ampl"=nan, "z∞ (V)"=0.0+0.0i, "4corners"={"z (-pi/2)"=9.277908004825974e-07+0.0007240755403629966i, "z(inf)"=2.6527949823343002e-05+0.0007477540585896028i, "z (pi/2)"=2.8494315967368497e-06+0.0007733542176124632i, "z center"=1.8886111986097237e-06+0.0007487148789877299i, "z(0)"=-2.2750727426123552e-05+0.000749675699385857i, "radius"=2.4658065287076567e-05}} {"z∞ (V)" format="%#_4p"; "Q" format="%#_4p"; "φ (rad)" format="%#_3p"; "Γ (Hz)" format="%#_5p"; "ω (Hz)" format="%#_9p"; "A (VHz)" format="%#_3p"}
  in  "save lor for later":bool
  in  "reset from basic":bool
  out "zi out Im (V)":dbl=8e-323 format="%#.8f"
  out "zi out Re (V)":dbl=1e-323 format="%#.8f"
  out "publish message":T4={"freq (Hz)"=6.9475337429379e-310, "gamma (Hz)"=0.9683990629933289, "Voltage (V)"=1e-323+8e-323i}
  out "zi out (V)":cdb=1e-323+8e-323i format="%#_5p"
  out "32bit integer":i32=5
  out "is publish loop stoped?":bool=TRUE
  out "window":T5={"cen (Hz)"=45496.74569300777, "win (Hz)"=29.962105514646385, "left (Hz)"=45481.76464025045, "right (Hz)"=45511.72674576509}
  out "running lorentzian out":T2={"A (VHz)"=0.009142510077437082, "ω (Hz)"=0.020119879746428596, "Γ (Hz)"=0.8109571797025381, "φ (rad)"=2.007511093178386, "Q"=0.02481003960506107, "Norm  Ampl"=nan, "z∞ (V)"=0.018500144394306906-0.0037766698823995634i, "4corners"={"z (-pi/2)"=0.023947397893225086+0.01120736437940613i, "z(inf)"=0.018500144394306906-0.0037766698823995634i, "z (pi/2)"=0.0334841786561126-0.009223923381317745i, "z center"=0.028715788274668842+0.0009917204990441924i, "z(0)"=0.03893143215503078+0.005760110880487949i, "radius"=0.011273727277179521}} {"z∞ (V)" format="%#_4p"; "Q" format="%#_4p"; "φ (rad)" format="%#_3p"; "Γ (Hz)" format="%#_5p"; "ω (Hz)" format="%#_9p"; "A (VHz)" format="%#_3p"}
  in  "lorentzian -- hist":T2={"A (VHz)"=0.00200421395131866, "ω (Hz)"=46345.85168996005, "Γ (Hz)"=30.48500465115163, "φ (rad)"=-1.4946726575691582, "Q"=1520.2835695880153, "Norm  Ampl"=nan, "z∞ (V)"=3.628480178228017e-06+0.00013828619430891303i, "4corners"={"z (-pi/2)"=-6.692524185707827e-05+0.0001988401926309779i, "z(inf)"=3.628480178228017e-06+0.00013828619430891303i, "z (pi/2)"=-5.692551814383685e-05+6.773247227360675e-05i, "z center"=-6.192538000045756e-05+0.00013328633245229232i, "z(0)"=-0.00012747924017914312+0.00012828647059567161i, "radius"=6.574425604501088e-05}} {"z∞ (V)" format="%#_4p"; "Q" format="%#_4p"; "φ (rad)" format="%#_3p"; "Γ (Hz)" format="%#_5p"; "ω (Hz)" format="%#_9p"; "A (VHz)" format="%#_3p"}
  out "slow f (Hz)":dbl=6.9475337429379e-310 format="%#.11f"
  out "slow G (Hz)":dbl=0.9683990629933289 format="%#.4f"
  in  "pll engine pair IN":T6
  out "static lorentzian out":T2 {"z∞ (V)" format="%#_4p"; "Q" format="%#_4p"; "φ (rad)" format="%#_3p"; "Γ (Hz)" format="%#_5p"; "ω (Hz)" format="%#_9p"; "A (VHz)" format="%#_3p"}
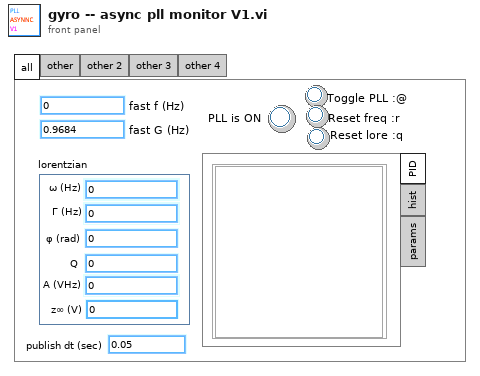
[diagram p1: front panel]
types:
  T1 = enum32{"all", "other", "other 2", "other 3", "other 4"}
  T2 = typedef "lorentzian.ctl" = cluster{"A (VHz)":dbl, "ω (Hz)":dbl, "Γ (Hz)":dbl, "φ (rad)":dbl, "Q":dbl, "Norm  Ampl":dbl, "z∞ (V)":cdb, "4corners":T3}
  T3 = typedef "circle corners.ctl" = cluster{"z (-pi/2)":cdb, "z(inf)":cdb, "z (pi/2)":cdb, "z center":cdb, "z(0)":cdb, "radius":dbl}
  T4 = cluster{"freq (Hz)":dbl, "gamma (Hz)":dbl, "Voltage (V)":cdb}
  T5 = typedef "show-win- control.ctl" = cluster{"cen (Hz)":dbl, "win (Hz)":dbl, "left (Hz)":dbl, "right (Hz)":dbl}
  T6 = typedef "server talk-to-back pair.ctl" = cluster{"talkback event":refnum<user-event>, "talkto event":refnum<user-event>}
  T7 = typedef "interpolation state - complex.ctl" = cluster{"requested size":i32, "Array":cdb[], "actual number of elements":i32}
  T8 = typedef "agregator -- action.ctl" = enum16{"append", "interpolate", "empty!", "force", "init", "scale", "read last"}
  T9 = typedef "launch items list.ctl" = enum16{"source", "pll engine", "pll monitor", "sweeper engine", "sweeper monitor", "fitter"}
  T10 = typedef "que event bag action.ctl" = enum16{"check", "add", "init", "keys", "values"}
  T11 = typedef "pll internal user event action.ctl" = enum16{"gear pll engine", "start pll async", "stop pll async", "toggle pll async", "gear sweeper", "start sweeper", "stop sweeper", "toggle sweeper", "accept frequency", "reset lorentzian", "accept lorentzian", "update cursors", "pause pll", "unpause pll", "void", "exit", "gear sweeper monitor", "gear sweeper engine", "gear fitter", "gear sourcer", "gear pll monitor"}
  T12 = typedef "interpolation state - real.ctl" = cluster{"Array ":dbl[], "actual size":i32, "requested size":i32}
  T13 = typedef "publisher action.ctl" = enum16{"set", "get", "init", "check"}
  T14 = typedef "server talkto message type.ctl" = cluster{"message":enum16{"stop", "start", "update pars", "update request", "new", "launch", "exit", "get", "reset", "pause", "unpause"}}
  T15 = typedef "four-corner circle transformation.ctl" = enum16{"z(c) z(inf)", "z(c) z(zero)", "fix phase", "calculate lorentzian", "z(0) z(+-pi/2)", "shift to zcenter", "to  canonical", "get canonical phase", "get4corners", "update lorentzian -- from z0", "fake gamma normal", "fake gamma heat", "calculate complex slope", "get f0 given f and phi"}
  T16 = typedef "cursor action.ctl" = enum16{"range", "read", "write", "check", "zoom out", "smart zoom out", "zoom to aspect ratio 1", "zoom to win", "zoom out 20%", "zoom in 20%", "-empty", "smart zoom out&aspect", "move range left 20%", "move range right 20%", "move range up 20%", "move range down 20%", "zoom to X win", "zoom to Y win", "zoom out X", "zoom out Y", "zoom in X", "zoom in Y", "check plot scale", "set plot color", "set Xlabel", "set Ylabel", "set cursor color"}
  T17 = typedef "eventvkey.ctl" = enum16{"ASCII", "Enter", "Return", "Shift", "Ctrl", "Alt", "Cmd", "Opt", "Caps", "NumLock", "Clear", "Break", "Up", "Down", "Left", "Right", "Insert", "Delete", "Home", "End", "PageUp", "PageDown", "Escape", "Help", "Pause", "ScrollLock", "F1", "F2", "F3", "F4", "F5", "F6", "F7", "F8", "F9", "F10", "F11", "F12", "F13", "F14", "F15", "F16", "F17", "F18", "F19", "F20", "F21", "F22", "F23", "F24", "Play", "VolumeUp", "VolumeDown", "Mute", "Two Byte Char"}
  T18 = typedef "pll talkback data type.ctl" = cluster{"ω (Hz)":dbl, "G (Hz)":dbl, "V (V)":cdb, "overlimit ?":bool, "running lorentzian out":T2, "static lorentzian out":T2}
  T19 = enum16{"stop", "start", "update pars", "update request", "new", "launch", "exit", "get", "reset", "pause", "unpause"}
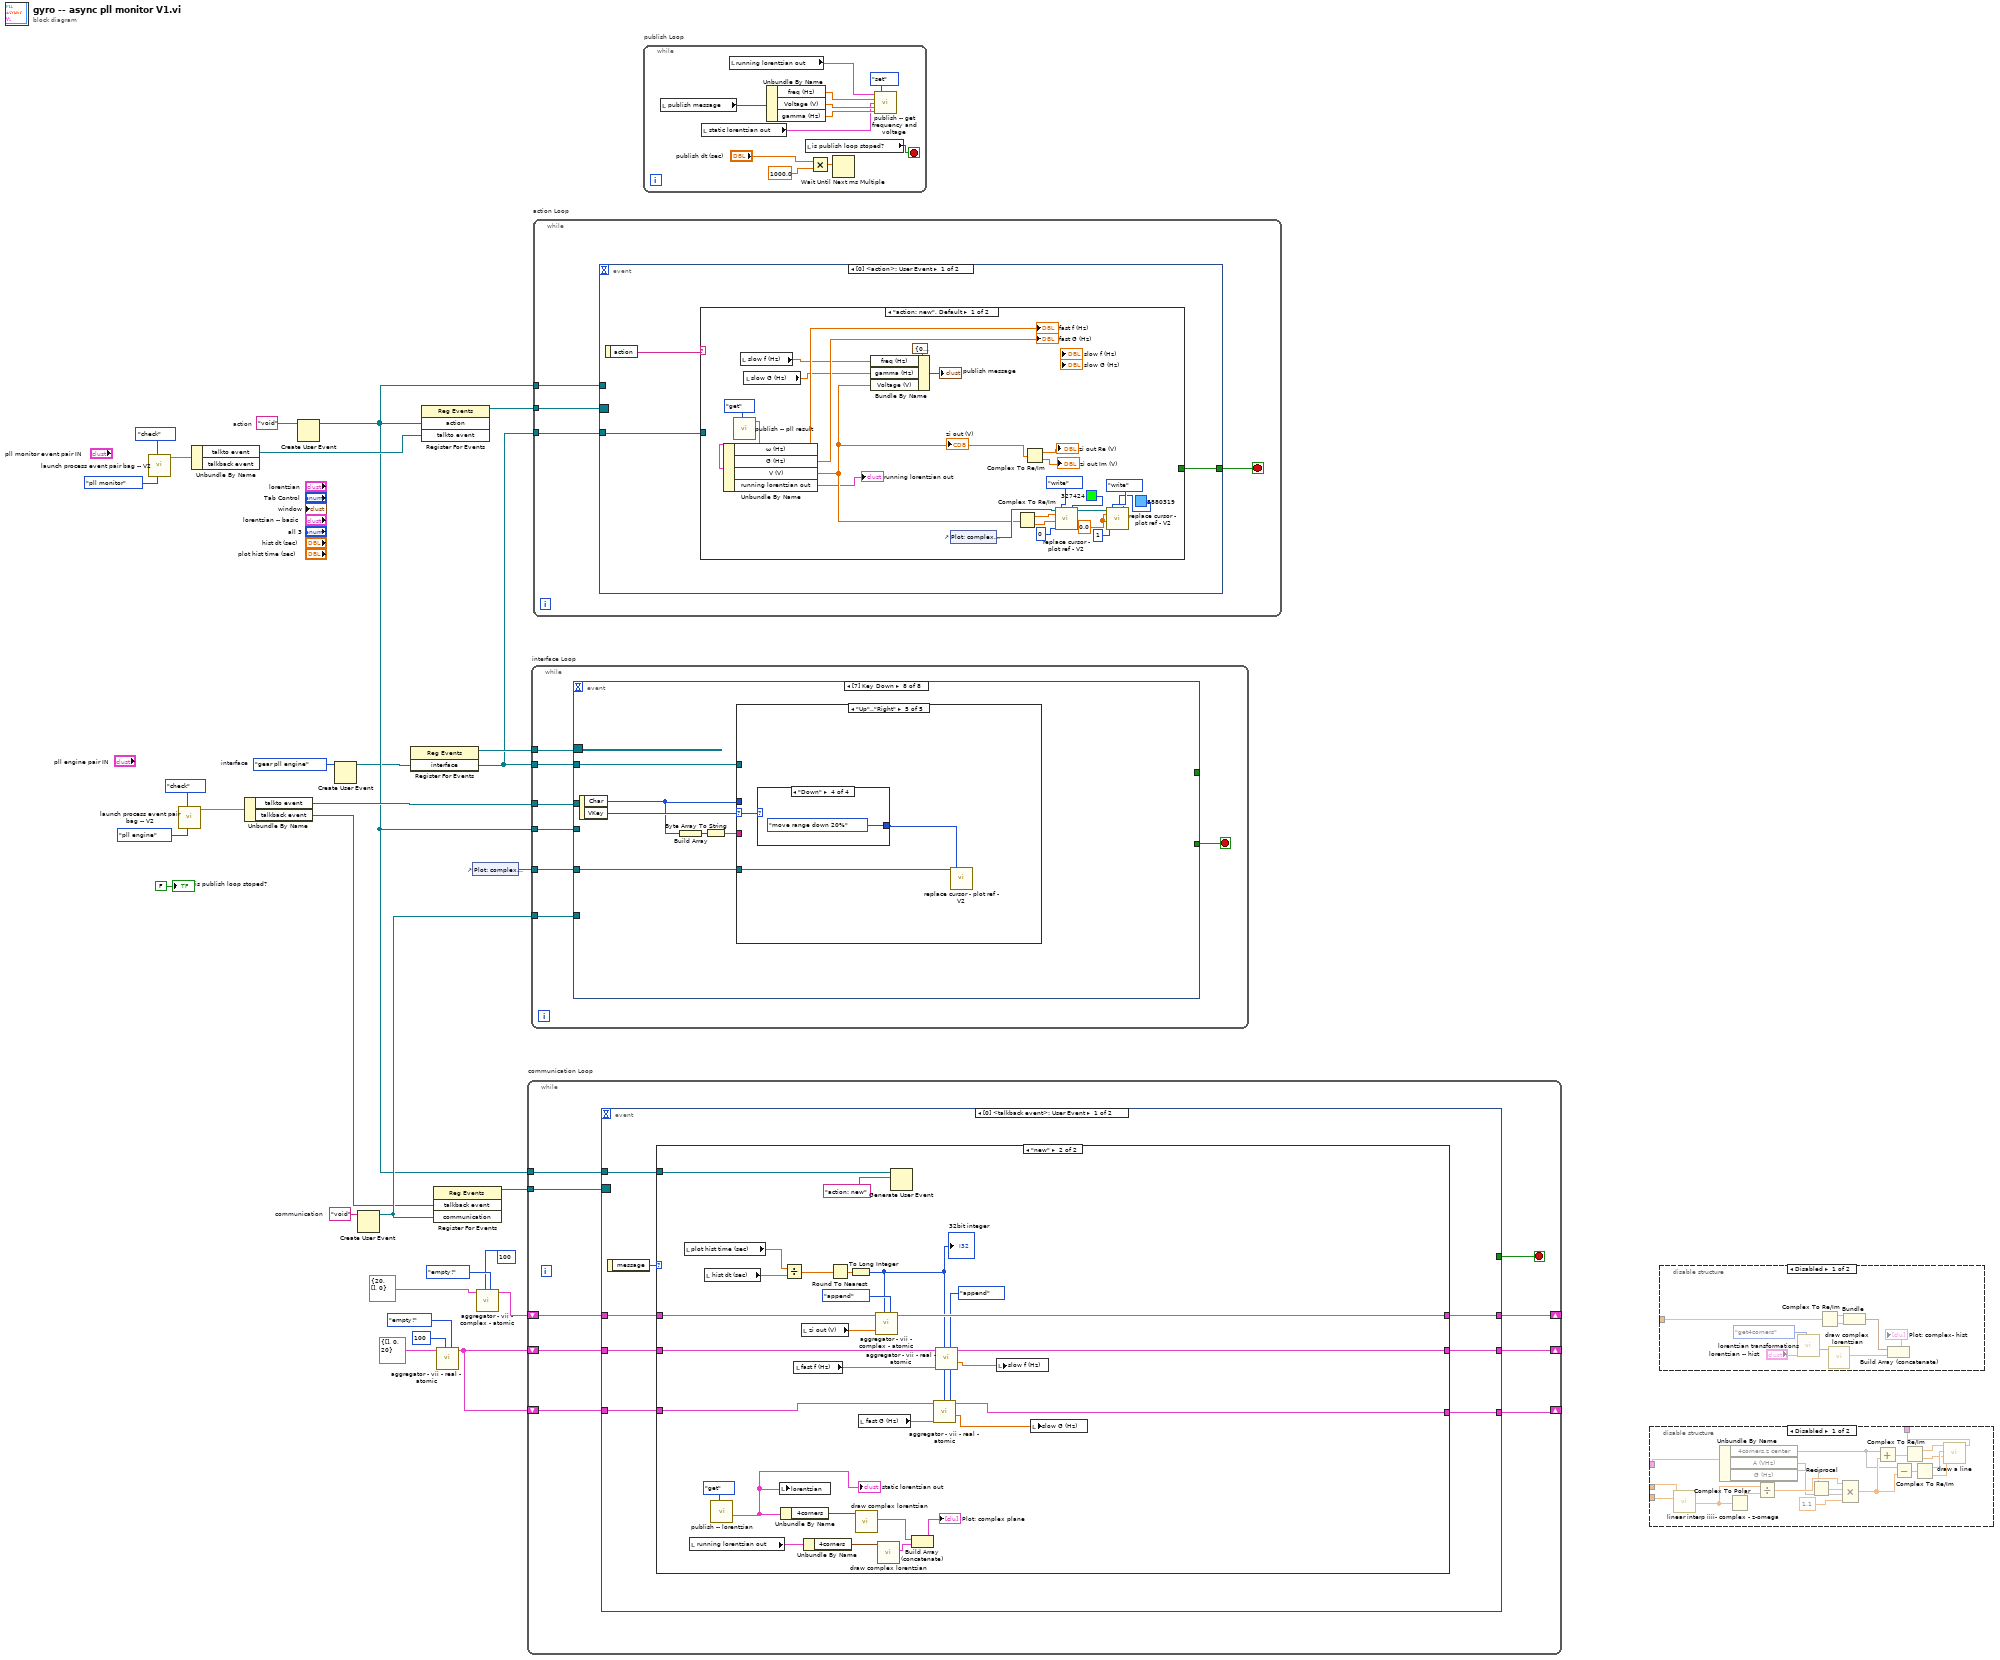
[diagram p0: block diagram]
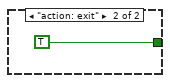
[diagram p4: hidden frame]
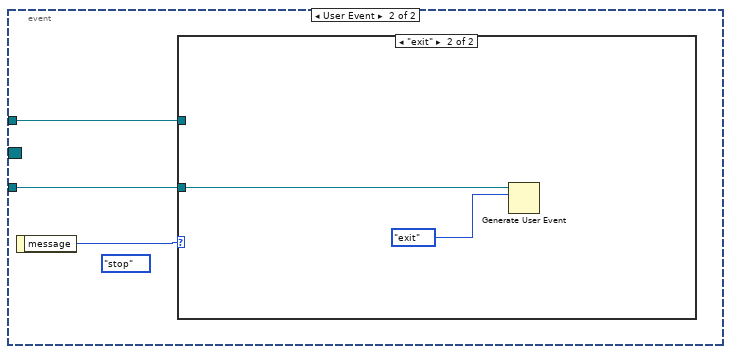
[diagram p5: hidden frame]
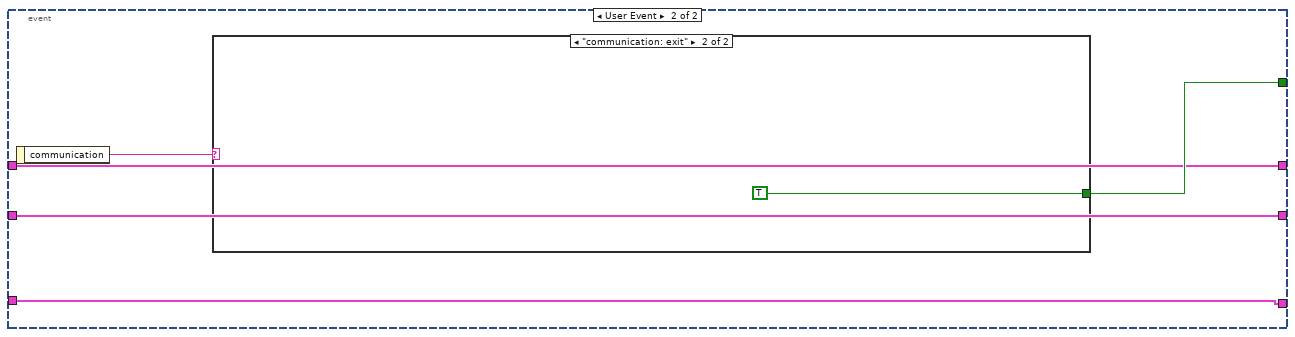
[diagram p8: hidden frame]
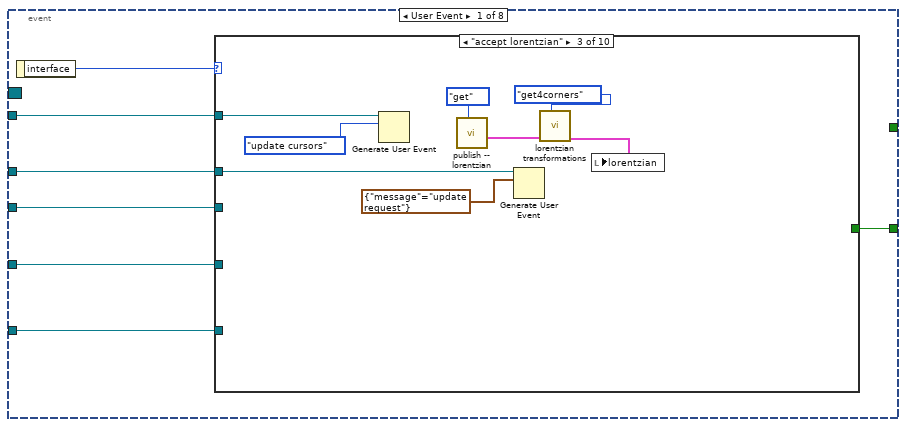
[diagram p10: hidden frame]
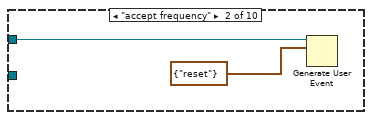
[diagram p12: hidden frame]
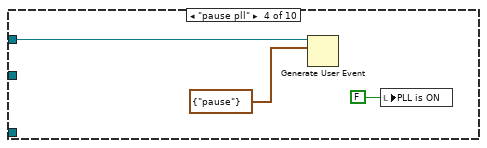
[diagram p13: hidden frame]
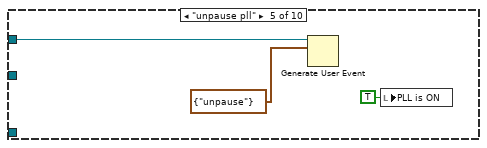
[diagram p14: hidden frame]
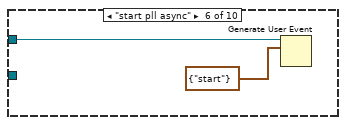
[diagram p15: hidden frame]
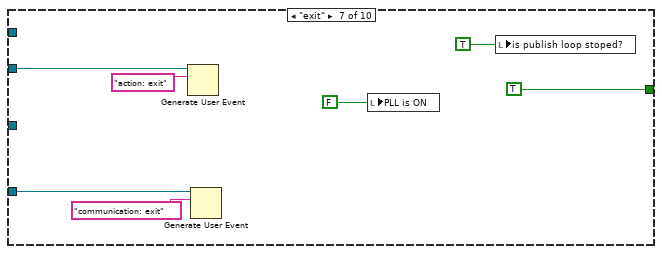
[diagram p16: hidden frame]
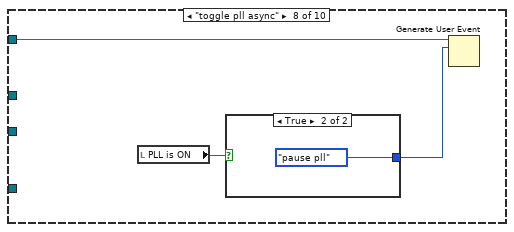
[diagram p17: hidden frame]
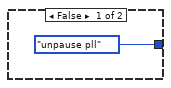
[diagram p18: hidden frame]
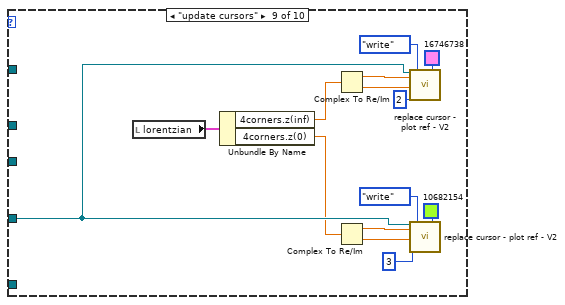
[diagram p19: hidden frame]
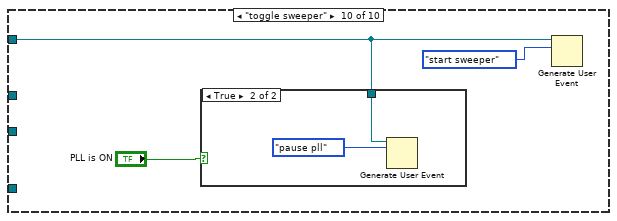
[diagram p20: hidden frame]
diagram:
  w18 = "void"  # communication
  w20 = "void"  # action
  w22 = pll_internal_user_event_action."gear pll engine"  # interface
  n1 = call "launch process event pair bag -- V2.vi"("launch item"=launch_items_list."pll monitor" ("launch items"), "bag action"=que_event_bag_action."check") -> ("event pair OUT"=w6:T6)  [unwired: 7 in, 2 out]
  n2 = call "launch process event pair bag -- V2.vi"("launch item"=launch_items_list."pll engine" ("launch items"), "bag action"=que_event_bag_action."check") -> ("event pair OUT"=w11:T6)  [unwired: 7 in, 2 out]
  n3 = Unbundle By Name(w6) -> ("talkto event"=w14:refnum<user-event>)  [unwired: 1 out]
  n4 = Unbundle By Name(w11) -> ("talkto event"=w16:refnum<user-event>, "talkback event"=w15:refnum<user-event>)
  n5 = Create User Event(user event datatype=w20) -> (user event=w13:refnum<user-event>)  [unwired: 1 in, 1 out]
  n6 = Create User Event(user event datatype=w22) -> (user event=w12:refnum<user-event>)  [unwired: 1 in, 1 out]
  n7 = Create User Event(user event datatype=w18) -> (user event=w17:refnum<user-event>)  [unwired: 1 in, 1 out]
  n8 = register-events(w12) -> (reference out=w28:refnum<event-registration>)  [unwired: 2 in, 1 out]
  n9 = register-events(w13, w14) -> (reference out=w19:refnum<event-registration>)  [unwired: 2 in, 1 out]
  n10 = register-events(w15, w17) -> (reference out=w24:refnum<event-registration>)  [unwired: 2 in, 1 out]
  n11 = call "aggregator - vii - real - atomic.vi"("aggregator action"=agregator_--_action."empty!", "requested size"=100, "state IN"=T12 {"Array "=[], "actual size"=0, "requested size"=20}) -> ("state OUT"=w5:T12)  [unwired: 5 in, 3 out]
  n12 = control-ref of="Plot: complex plane"() -> (w23:refnum<vi>)
  n13 = call "aggregator - vii - complex - atomic.vi"("aggregator action"=agregator_--_action."empty!", "requested size"=100, "state IN"=T7 {"requested size"=20, "Array"=[], "actual number of elements"=0}) -> ("state OUT"=w3:T7)  [unwired: 5 in, 3 out]
  n14 = while "communication Loop" {
    shift-right: [w34] -> _
    shift-left: w3 -> [w37]
    shift-right: [w35] -> _
    shift-left: w5 -> [w36]
    tunnel: w24 -> [w33]
    tunnel: w13 -> [w32]
    shift-right: [w30] -> _
    shift-left: w5 -> [w29]
    stop <- w31 stop-if-true
    n15 = event shown="[0] <talkback event>: User Event" {
      selector: w33 -> [_ _]
      dyn-events: _ -> [_ _]
      timeout: _ -> [_ _]
      tunnel: w37 -> [w45 w79]
      tunnel: w36 -> [w44 w78]
      tunnel: [w43 w78] -> w35
      tunnel: [w42 w79] -> w34
      tunnel: w32 -> [w40 _]
      tunnel: [_ w80] -> w31
      tunnel: [w39 w77] -> w30
      tunnel: w29 -> [w38 w77]
      event User Event {
        n16 = event-data() -> ("message"=w41:enum16{"new", "void"})  [unwired: 1 in]
        n17 = case shown="\"new\"" w41 {
          tunnel: w45 -> [w48 w76]
          tunnel: w44 -> [w47 w74]
          tunnel: [w47 w73] -> w43
          tunnel: [w48 w70] -> w42
          tunnel: w40 -> [_ w67]
          tunnel: [w46 w53] -> w39
          tunnel: w38 -> [w46 w52]
          frame "void", Default {
          }
          frame "new" {
            w54 = agregator_--_action."append" ("aggregator action")
            n18 = local read "plot hist time (sec)"() -> (w68:dbl)
            n19 = local read "running lorentzian out"() -> (w57:T2)
            n20 = local read "hist dt (sec)"() -> (w69:dbl)
            n21 = call "publish -- lorentzian.vi"("publisher action"=publisher_action."get") -> ("lorentzian OUT"=w56:T2)  [unwired: 10 in]
            "static lorentzian out" <- w56
            n22 = local write "lorentzian"(w56) -> ()
            n23 = Unbundle By Name(w56) -> ("4corners"=w62:T3)
            n24 = Divide(x=w68, y=w69) -> (x/y=w72:dbl)
            n25 = local read "fast f (Hz)"() -> (w65:dbl)
            n26 = local read "zi out (V)"() -> (w64:cdb)
            n27 = Unbundle By Name(w57) -> ("4corners"=w61:T3)
            n28 = Round To Nearest(number=w72) -> (nearest integer value=w71:dbl)
            n29 = To Long Integer(number=w71) -> (32bit integer=w55:i32)
            "32bit integer" <- w55
            n30 = call "draw complex lorentzian.vi"("4 corners"=w62) -> ("fancy circles"=w60:cluster{dbl[], dbl[]}[])  [unwired: 10 in]
            n31 = local read "fast G (Hz)"() -> (w51:dbl)
            n32 = call "aggregator - vii - complex - atomic.vi"("aggregator action"=agregator_--_action."append", "requested size"=w55, "number"=w64, "state IN"=w76) -> ("state OUT"=w70:T7)  [unwired: 4 in, 3 out]
            n33 = call "draw complex lorentzian.vi"("4 corners"=w61) -> ("fancy circles"=w59:cluster{dbl[], dbl[]}[])  [unwired: 10 in]
            n34 = Generate User Event(user event=w67, event data cluster="action: new" ("event data")) -> ()  [unwired: 2 in, 2 out]
            n35 = Build Array (concatenate)(w60, w59) -> (→"Plot: complex plane":cluster{dbl[], dbl[]}[])
            n36 = call "aggregator - vii - real - atomic.vi"("aggregator action"=w54, "requested size"=w55, "number"=w51, "state IN"=w52) -> ("interp average"=w50:dbl, "state OUT"=w53:T12)  [unwired: 4 in, 2 out]
            n37 = call "aggregator - vii - real - atomic.vi"("aggregator action"=w54, "requested size"=w55, "number"=w65, "state IN"=w74) -> ("interp average"=w49:dbl, "state OUT"=w73:T12)  [unwired: 4 in, 2 out]
            n38 = local write "slow f (Hz)"(w49) -> ()
            n39 = local write "slow G (Hz)"(w50) -> ()
          }
        }
      }
      event User Event {
        n40 = event-data() -> ("communication"=w81:string)  [unwired: 1 in]
        n41 = case shown="\"communication: exit\"" w81 {
          tunnel: [_ TRUE] -> w80
          frame "void", Default {
          }
          frame "communication: exit" {
          }
        }
      }
    }
  }
  n42 = while "interface Loop" {
    tunnel: w28 -> [w89]
    tunnel: w12 -> [w88]
    tunnel: w23 -> [w87]
    tunnel: w16 -> [w86]
    tunnel: w13 -> [w84]
    tunnel: w17 -> [w83]
    stop <- w85 stop-if-true
    n43 = event shown="[7] Key Down" {
      selector: w89 -> [_ _ _ _ _ _ _ _]
      dyn-events: _ -> [_ _ _ _ _ _ _ _]
      timeout: _ -> [_ _ _ _ _ _ _ _]
      tunnel: [_ "Toggle PLL :@" _ "Reset freq :r" "Reset lore :q" "reset from basic" "save lor for later" _] -> _
      tunnel: w88 -> [w94 w148 _ w183 w186 _ _ w196]
      tunnel: w87 -> [w95 _ w154 _ _ _ _ w195]
      tunnel: w86 -> [w93 _ _ _ _ _ _ _]
      tunnel: [w92 _ _ _ _ _ _ _] -> w85
      tunnel: w84 -> [w91 _ _ _ _ _ _ _]
      tunnel: w83 -> [w90 _ _ _ _ _ _ _]
      event User Event {
        n44 = event-data() -> ("interface"=w96:T11)  [unwired: 1 in]
        n45 = case shown="\"accept lorentzian\"" w96 {
          tunnel: w95 -> [_ _ _ _ _ _ _ _ w140 _]
          tunnel: w94 -> [_ _ w101 _ _ _ _ w124 _ w142]
          tunnel: w93 -> [_ w98 w106 w109 w112 w113 _ _ _ _]
          tunnel: [_ _ _ _ _ _ TRUE _ _ _] -> w92
          tunnel: w91 -> [_ _ _ _ _ _ w118 _ _ _]
          tunnel: w90 -> [_ _ _ _ _ _ w115 _ _ _]
          frame "void", Default {
          }
          frame "accept frequency" {
            n46 = Generate User Event(user event=w98, event data cluster=T14 {"message"=enum."reset"} ("event data")) -> ()  [unwired: 2 in, 2 out]
          }
          frame "accept lorentzian" {
            n47 = Generate User Event(user event=w101, event data cluster=pll_internal_user_event_action."update cursors" ("event data")) -> ()  [unwired: 2 in, 2 out]
            n48 = call "publish -- lorentzian.vi"("publisher action"=publisher_action."get") -> ("lorentzian OUT"=w105:T2)  [unwired: 10 in]
            n49 = Generate User Event(user event=w106, event data cluster=T14 {"message"=enum."update request"} ("event data")) -> ()  [unwired: 2 in, 2 out]
            n50 = call "lorentzian transformations.vi"("4 corner circle transformation"=four-corner_circle_transformation."get4corners", "lorentzian in"=w105) -> ("lorentzian out"=w104:T2)  [unwired: 6 in, 3 out]
            n51 = local write "lorentzian"(w104) -> ()
          }
          frame "pause pll" {
            n52 = Generate User Event(user event=w109, event data cluster=T14 {"message"=enum."pause"} ("event data")) -> ()  [unwired: 2 in, 2 out]
            n53 = local write "PLL is ON"(FALSE ("PLL ON")) -> ()
          }
          frame "unpause pll" {
            n54 = Generate User Event(user event=w112, event data cluster=T14 {"message"=enum."unpause"} ("event data")) -> ()  [unwired: 2 in, 2 out]
            n55 = local write "PLL is ON"(TRUE ("PLL ON")) -> ()
          }
          frame "start pll async" {
            n56 = Generate User Event(user event=w113, event data cluster=T14 {"message"=enum."start"} ("event data")) -> ()  [unwired: 2 in, 2 out]
          }
          frame "exit" {
            n57 = Generate User Event(user event=w118, event data cluster="action: exit" ("event data")) -> ()  [unwired: 2 in, 2 out]
            n58 = Generate User Event(user event=w115, event data cluster="communication: exit" ("event data")) -> ()  [unwired: 2 in, 2 out]
            n59 = local write "PLL is ON"(FALSE ("PLL ON")) -> ()
            n60 = local write "is publish loop stoped?"(TRUE ("Stoped?")) -> ()
          }
          frame "toggle pll async" {
            n61 = local read "PLL is ON"() -> (w123:bool)
            n62 = case shown="True" w123 {
              tunnel: [pll_internal_user_event_action."unpause pll" ("event data") pll_internal_user_event_action."pause pll" ("event data")] -> w122
              frame False {
              }
              frame True {
              }
            }
            n63 = Generate User Event(user event=w124, event data cluster=w122) -> ()  [unwired: 2 in, 2 out]
          }
          frame "update cursors" {
            n64 = local read "lorentzian"() -> (w127:T2)
            n65 = Unbundle By Name(w127) -> ("4corners.z(inf)"=w135:cdb, "4corners.z(0)"=w128:cdb)
            n66 = Complex To Re/Im(x + iy=w135) -> (x=w137:dbl, y=w136:dbl)
            n67 = Complex To Re/Im(x + iy=w128) -> (x=w131:dbl, y=w130:dbl)
            n68 = call "replace cursor - plot ref - V2.vi"("Plot ref in"=w140, "new X"=w137, "new  Y"=w136, "cursor index"=2, "cursor action"=cursor_action."write", "Color Box"=u32 16746738) -> ()  [unwired: 10 in, 4 out]
            n69 = call "replace cursor - plot ref - V2.vi"("Plot ref in"=w140, "new X"=w131, "new  Y"=w130, "cursor index"=3, "cursor action"=cursor_action."write", "Color Box"=u32 10682154) -> ()  [unwired: 10 in, 4 out]
          }
          frame "toggle sweeper" {
            n70 = case shown="True" "PLL is ON" {
              tunnel: w142 -> [_ w144]
              frame False {
              }
              frame True {
                n71 = Generate User Event(user event=w144, event data cluster=pll_internal_user_event_action."pause pll" ("event data")) -> ()  [unwired: 2 in, 2 out]
              }
            }
            n72 = Generate User Event(user event=w142, event data cluster=pll_internal_user_event_action."start sweeper" ("event data")) -> ()  [unwired: 2 in, 2 out]
          }
        }
      }
      event "Toggle PLL :@": Value Change {
        w146 = pll_internal_user_event_action."toggle pll async"  # event data
        n73 = event-data() -> ()  [unwired: 1 in, 1 out]
        n74 = Generate User Event(user event=w148, event data cluster=w146) -> ()  [unwired: 2 in, 2 out]
      }
      event "Plot: complex plane": Cursor Move {
        n75 = event-data() -> ("CursIdx"=w153:i32)  [unwired: 1 in]
        n76 = local read "lorentzian"() -> (w152:T2)
        n77 = case shown="2" w153 {
          selector: w153 -> [_ w166 w176]
          tunnel: w154 -> [_ w160 w175]
          tunnel: w152 -> [w155 w156 w174]
          tunnel: [w155 w157 w171] -> w150
          frame 0, Default {
          }
          frame 2 {
            n78 = call "replace cursor - plot ref - V2.vi"("Plot ref in"=w160, "cursor index"=w166, "cursor action"=cursor_action."read") -> ("read X"=w168:dbl, "read Y"=w169:dbl)  [unwired: 13 in, 2 out]
            n79 = Re/Im To Complex(1:w169, 2:w168) -> (0:w167:cdb)
            n80 = Bundle By Name(cluster=w156, "z∞ (V)"=w167) -> (w165:T2)
            n81 = call "lorentzian transformations.vi"("4 corner circle transformation"=four-corner_circle_transformation."get4corners", "lorentzian in"=w165) -> ("lorentzian out"=w157:T2)  [unwired: 6 in, 3 out]
            n82 = Unbundle By Name(w157) -> ("4corners.z(0)"=w163:cdb)
            n83 = Complex To Re/Im(x + iy=w163) -> (x=w162:dbl, y=w161:dbl)
            n84 = call "replace cursor - plot ref - V2.vi"("Plot ref in"=w160, "new X"=w162, "new  Y"=w161, "cursor index"=3, "cursor action"=cursor_action."write") -> ()  [unwired: 11 in, 4 out]
          }
          frame 3 {
            n85 = call "replace cursor - plot ref - V2.vi"("Plot ref in"=w175, "cursor index"=w176, "cursor action"=cursor_action."read") -> ("read X"=w178:dbl, "read Y"=w179:dbl)  [unwired: 13 in, 2 out]
            n86 = Re/Im To Complex(1:w179, 2:w178) -> (0:w177:cdb)
            n87 = Bundle By Name(cluster=w174, "4corners.z(0)"=w177) -> (w173:T2)
            n88 = call "lorentzian transformations.vi"("4 corner circle transformation"=four-corner_circle_transformation."update lorentzian -- from z0", "lorentzian in"=w173) -> ("lorentzian out"=w171:T2)  [unwired: 6 in, 3 out]
          }
        }
        n89 = call "lorentzian transformations.vi"("4 corner circle transformation"=four-corner_circle_transformation."get4corners", "lorentzian in"=w150) -> ("lorentzian out"=w149:T2)  [unwired: 6 in, 3 out]
        n90 = local write "lorentzian"(w149) -> ()
      }
      event "Reset freq :r": Value Change {
        n91 = event-data() -> ()  [unwired: 1 in, 1 out]
        n92 = Generate User Event(user event=w183, event data cluster=pll_internal_user_event_action."accept frequency" ("event data")) -> ()  [unwired: 2 in, 2 out]
      }
      event "Reset lore :q": Value Change {
        n93 = event-data() -> ()  [unwired: 1 in, 6 out]
        n94 = Generate User Event(user event=w186, event data cluster=pll_internal_user_event_action."accept lorentzian" ("event data")) -> ()  [unwired: 2 in, 2 out]
      }
      event "reset from basic": Value Change {
        n95 = event-data() -> ()  [unwired: 1 in, 6 out]
        n96 = local read "lorentzian -- basic"() -> (w188:T2)
        n97 = call "lorentzian transformations.vi"("4 corner circle transformation"=four-corner_circle_transformation."get4corners", "lorentzian in"=w188) -> ("lorentzian out"=w187:T2)  [unwired: 6 in, 3 out]
        n98 = local write "lorentzian"(w187) -> ()
      }
      event "save lor for later": Value Change {
        n99 = event-data() -> ()  [unwired: 1 in, 6 out]
        n100 = local read "lorentzian"() -> (w192:T2)
        n101 = call "lorentzian transformations.vi"("4 corner circle transformation"=four-corner_circle_transformation."get4corners", "lorentzian in"=w192) -> ("lorentzian out"=w191:T2)  [unwired: 6 in, 3 out]
        n102 = local write "lorentzian -- basic"(w191) -> ()
      }
      event Key Down {
        n103 = event-data() -> ("Char"=w198:i16, "VKey"=w200:T17)  [unwired: 1 in]
        n104 = Build Array(w198) -> (w199:i16[])
        n105 = Byte Array To String(unsigned byte array=w199) -> (string=w197:string)
        n106 = case shown="\"Up\"..\"Right\"" w200 {
          selector: w200 -> [_ _ _ _ w222]
          tunnel: w198 -> [_ _ _ _ _]
          tunnel: w197 -> [w203 _ _ _ _]
          tunnel: w196 -> [w202 _ _ _ _]
          tunnel: w195 -> [w201 _ _ _ w221]
          frame "ASCII", Default {
            n107 = case shown="\"<\", \">\", \"?\", \"A\", \"z\"" w203 {
              selector: w203 -> [_ w205 _ _ _ _ _]
              tunnel: w202 -> [_ _ w213 _ w215 w217 w219]
              tunnel: w201 -> [_ w204 _ _ _ _ _]
              frame "0", Default {
              }
              frame "<", ">", "?", "A", "z" {
                n108 = case shown="\"A\"" w205 {
                  tunnel: [cursor_action."zoom out 20%" ("cursor action") cursor_action."zoom in 20%" ("cursor action") cursor_action."smart zoom out&aspect" ("cursor action") cursor_action."smart zoom out" ("cursor action") cursor_action."zoom to aspect ratio 1" ("cursor action")] -> w206
                  frame ">" {
                  }
                  frame "<" {
                  }
                  frame "?" {
                  }
                  frame "A" {
                  }
                  frame "z", Default {
                  }
                }
                n109 = call "replace cursor - plot ref - V2.vi"("Plot ref in"=w204, "cursor action"=w206) -> ()  [unwired: 14 in, 4 out]
              }
              frame "r" {
                (unwired) "reset frequency" ("event data")
                n110 = Generate User Event(user event=w213, event data cluster=pll_internal_user_event_action."accept frequency" ("event data")) -> ()  [unwired: 2 in, 2 out]
              }
              frame "'", ";", "[", "]", "{", "}" {
              }
              frame "@" {
                (unwired) "toggle PLL" ("event data")
                n111 = Generate User Event(user event=w215, event data cluster=pll_internal_user_event_action."toggle pll async" ("event data")) -> ()  [unwired: 2 in, 2 out]
              }
              frame "#" {
                (unwired) "(sweeper) sweep!" ("event data")
                n112 = Generate User Event(user event=w217, event data cluster=pll_internal_user_event_action."toggle sweeper" ("event data")) -> ()  [unwired: 2 in, 2 out]
              }
              frame "q" {
                (unwired) "reset lorentzian" ("event data")
                n113 = Generate User Event(user event=w219, event data cluster=pll_internal_user_event_action."accept lorentzian" ("event data")) -> ()  [unwired: 2 in, 2 out]
              }
            }
          }
          frame "Escape" {
          }
          frame "PageUp" {
          }
          frame "PageDown" {
          }
          frame "Up".."Right" {
            n114 = case shown="\"Down\"" w222 {
              tunnel: [cursor_action."move range right 20%" ("cursor action") cursor_action."move range left 20%" ("cursor action") cursor_action."move range up 20%" ("cursor action") cursor_action."move range down 20%" ("cursor action")] -> w220
              frame "Right", Default {
              }
              frame "Left" {
              }
              frame "Up" {
              }
              frame "Down" {
              }
            }
            n115 = call "replace cursor - plot ref - V2.vi"("Plot ref in"=w221, "cursor action"=w220) -> ()  [unwired: 14 in, 4 out]
          }
        }
      }
    }
  }
  n116 = while "action Loop" {
    tunnel: w19 -> [w230]
    tunnel: w13 -> [w228]
    tunnel: w12 -> [w227]
    stop <- w229 stop-if-true
    n117 = event shown="[0] <action>: User Event" {
      selector: w230 -> [_ _]
      dyn-events: _ -> [_ _]
      timeout: _ -> [_ _]
      tunnel: [w232 _] -> w229
      tunnel: w228 -> [_ w259]
      tunnel: w227 -> [w231 w258]
      event User Event {
        n118 = event-data() -> ("action"=w233:string)  [unwired: 1 in]
        n119 = case shown="\"action: new\", Default" w233 {
          tunnel: [_ TRUE] -> w232
          tunnel: w231 -> [_ _]
          frame "action: new", Default {
            w244 = 0.0 ("new X")
            n120 = call "publish -- pll result.vi"("publisher action"=publisher_action."get") -> ("pll result OUT"=w252:T18)  [unwired: 10 in]
            n121 = Unbundle By Name(w252) -> ("ω (Hz)"=→"fast f (Hz)":dbl, "G (Hz)"=→"fast G (Hz)":dbl, "V (V)"=w255:cdb, "running lorentzian out"=→"running lorentzian out":T2)
            "zi out (V)" <- w255
            n122 = local read "slow f (Hz)"() -> (w234:dbl)
            n123 = local read "slow G (Hz)"() -> (w235:dbl)
            n124 = Bundle By Name(cluster=T4 {"freq (Hz)"=0.0, "gamma (Hz)"=0.0, "Voltage (V)"=0.0+0.0i} ("publish message"), "freq (Hz)"=w234, "gamma (Hz)"=w235, "Voltage (V)"=w255) -> (→"publish message":T4)
            n125 = control-ref of="Plot: complex plane"() -> (w256:refnum<vi>)
            n126 = Complex To Re/Im(x + iy=w255) -> (x=w248:dbl, y=w247:dbl)
            n127 = Complex To Re/Im(x + iy=w255) -> (x=→"zi out Re (V)":dbl, y=→"zi out Im (V)":dbl)
            n128 = call "replace cursor - plot ref - V2.vi"("Plot ref in"=w256, "new X"=w248, "new  Y"=w247, "cursor index"=0, "cursor action"=cursor_action."write", "Color Box"=u32 327424) -> ("Plot ref out"=w246:refnum<vi>)  [unwired: 10 in, 3 out]
            n129 = call "replace cursor - plot ref - V2.vi"("Plot ref in"=w246, "new X"=w244, "new  Y"=w244, "cursor index"=1, "cursor action"=cursor_action."write", "Color Box"=u32 5880319) -> ()  [unwired: 10 in, 4 out]
          }
          frame "action: exit" {
          }
        }
      }
      event User Event {
        (unwired) T19."stop" ("message")
        n130 = event-data() -> ("message"=w260:T19)  [unwired: 1 in]
        n131 = case shown="\"exit\"" w260 {
          tunnel: w259 -> [_ _]
          tunnel: w258 -> [_ w261]
          frame "stop", Default {
          }
          frame "exit" {
            n132 = Generate User Event(user event=w261, event data cluster=pll_internal_user_event_action."exit" ("event data")) -> ()  [unwired: 2 in, 2 out]
          }
        }
      }
    }
  }
  n133 = while "publish Loop" {
    stop <- w268 stop-if-true
    n134 = local read "publish message"() -> (w272:T4)
    n135 = local read "static lorentzian out"() -> (w263:T2)
    n136 = local read "running lorentzian out"() -> (w264:T2)
    n137 = Unbundle By Name(w272) -> ("freq (Hz)"=w271:dbl, "Voltage (V)"=w270:cdb, "gamma (Hz)"=w269:dbl)
    n138 = local read "is publish loop stoped?"() -> (w268:bool)
    n139 = Multiply(x="publish dt (sec)", y=1000.0) -> (x*y=w266:dbl)
    n140 = Wait Until Next ms Multiple(millisecond multiple=w266) -> ()  [unwired: 1 out]
    n141 = call "publish -- get frequency and voltage.vi"("running lorentzian in"=w264, "publisher action"=publisher_action."set", "freq IN (Hz)"=w271, "static lorentzian IN"=w263, "Voltage IN (V)"=w270, "gamma IN (Hz)"=w269) -> ()  [unwired: 5 in, 5 out]
  }
  n142 = disable-structure shown="Disabled" {
    disable-tunnel: _ -> [w292 _]
    disable-tunnel: _ -> [w291 _]
    disable-tunnel: [w276 _] -> _
    disable-tunnel: _ -> [w274 _]
    frame Disabled {
      n143 = call "linear interp iiii- complex - z-omega.vi"("z"=w292, "omega"=w291) -> ("slope"=w290:cdb)  [unwired: 5 in, 8 out]
      n144 = Unbundle By Name(w274) -> ("4corners.z center"=w275, "A (VHz)"=w285, "G (Hz)"=w287)
      n145 = Complex To Polar(r * e^(i*theta)=w290) -> (r=w289:dbl)  [unwired: 1 out]
      n146 = Divide(x=w290, y=w289) -> (x/y=w288:cdb)
      n147 = Reciprocal(x=w287) -> (1/x=w286:dbl)
      n148 = Compound Arithmetic op=MULTIPLY(w288, w286, w285, 1.1 ("value")) -> (w278:cdb)
      n149 = Add(x=w275, y=w278) -> (x+y=w284:cdb)
      n150 = Subtract(x=w275, y=w278) -> (x-y=w283:cdb)
      n151 = Complex To Re/Im(x + iy=w284) -> (x=w282:dbl, y=w280:dbl)
      n152 = Complex To Re/Im(x + iy=w283) -> (x=w281:dbl, y=w279:dbl)
      n153 = call "draw a line.vi"("y1"=w279, "y0"=w280, "x1"=w281, "x0"=w282) -> ("output cluster"=w276:cluster{dbl[], dbl[]})  [unwired: 7 in]
    }
    frame Enabled {
    }
  }
  n154 = disable-structure shown="Disabled" {
    disable-tunnel: _ -> [w293 _]
    frame Disabled {
      n155 = call "lorentzian transformations.vi"("4 corner circle transformation"=four-corner_circle_transformation."get4corners", "lorentzian in"="lorentzian -- hist") -> ("4corners our"=w297:T3)  [unwired: 6 in, 3 out]
      n156 = Complex To Re/Im(x + iy=w293) -> (x=w300:dbl, y=w299:dbl)
      n157 = call "draw complex lorentzian.vi"("4 corners"=w297) -> ("fancy circles"=w295:cluster{dbl[], dbl[]}[])  [unwired: 10 in]
      n158 = Bundle(w300, w299) -> (w301:cluster{dbl, dbl})  [unwired: 1 in]
      n159 = Build Array (concatenate)(w301, w295) -> (→"Plot: complex- hist":cluster{dbl[], dbl[]}[])
    }
    frame Enabled {
    }
  }
  "is publish loop stoped?" <- FALSE ("Stoped?")
